vi "uTransport_SendMsg.vi"(8 "error in (no error)":errorcluster, 10 "Msg":refnum<class "uMsg.lvclass">, 11 "uTransport in":refnum<class "uTransport.lvclass">) -> (0 "error out":errorcluster, 3 "uTransport out":refnum<class "uTransport.lvclass">)   [LabVIEW 2023, in "uLib.lvlib" / "uTransport.lvclass"]
doc: "Send a message to the transport.\n\nIf the message is not timestamped in itself and a value is not provided to the timestamp teminal on the connector pane, then the method automatically applies the current tick count as time stamp.\n\nIf a timestamp is wired to the copane, the timestamp in the uMsg is overwritten."
uses:
  uTransport.lvclass
  uMsg/uMsg/uMsg.lvclass
  uMsg/uMsg/uMsg.lvclass/uMsg.ctl
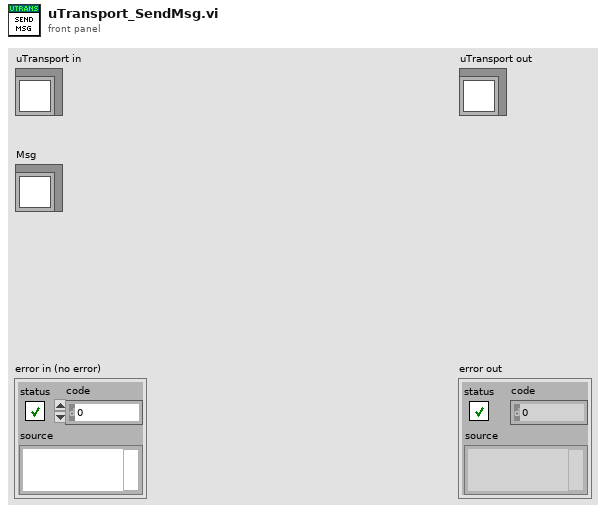
[diagram p1: front panel]
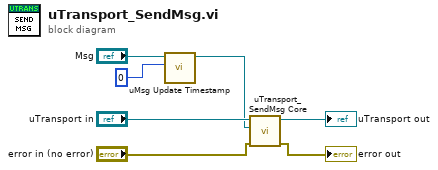
[diagram p0: block diagram]
diagram:
  n1 = call "uMsg Update Timestamp.vi"("Timestamp"=u32 0, "uMsg in"="Msg") -> ("uMsg out"=w2:refnum<class "uMsg.lvclass">)  [unwired: 8 in, 1 out]
  n2 = call-dynamic "uTransport_SendMsg Core.vi"("error in (no error)"="error in (no error)", "Msg"=w2, "uTransport in"="uTransport in") -> ("error out"=→"error out":errorcluster, "uTransport out"=→"uTransport out":refnum<class "uTransport.lvclass">)  [unwired: 7 in]
